vi "Set Exp to test_Charge Transfer.vi"(0 "Test Information":T3={"Exp Name"="Cold Switching", "Lot"="0233A", "Wafer"="15", "Die Type"="L22", "Die X "="6", "Die Y"="8", "Exp"="1", "Die X_Y"="8"}, 5 "Experiments":T2={"Exp 1"={"P2_Sweep_Stop_V"=36.0, "Res Threshold"=1.0, "P2_Sweep_Start_V"=36.0, "P2_Sweep_Step_V"=1.0, "Experiment Name"="", "P1_Sweep_Start_V"=36.0, "P1_Sweep_Step_V"=1.0, "P1_Peak_Array"=[]}, "Exp 2"={"P2_Sweep_Stop_V"=36.0, "Res Threshold"=1.0, "P2_Sweep_Start_V"=36.0, "P2_Sweep_Step_V"=1.0, "Experiment Name"="", "P1_Sweep_Start_V"=36.0, "P1_Sweep_Step_V"=1.0, "P1_Peak_Array"=[]}, "Exp 3"={"P2_Sweep_Stop_V"=36.0, "Res Threshold"=1.0, "P2_Sweep_Start_V"=36.0, "P2_Sweep_Step_V"=1.0, "Experiment Name"="", "P1_Sweep_Start_V"=36.0, "P1_Sweep_Step_V"=1.0, "P1_Peak_Array"=[]}, "Exp 4"={"P2_Sweep_Stop_V"=36.0, "Res Threshold"=1.0, "P2_Sweep_Start_V"=36.0, "P2_Sweep_Step_V"=1.0, "Experiment Name"="", "P1_Sweep_Start_V"=36.0, "P1_Sweep_Step_V"=1.0, "P1_Peak_Array"=[]}}, 11 "Error In":errorcluster) -> (4 "Selected Exp Settings":T1={"P2_Sweep_Stop_V"=36.0, "Res Threshold"=1.0, "P2_Sweep_Start_V"=36.0, "P2_Sweep_Step_V"=1.0, "Experiment Name"="", "P1_Sweep_Start_V"=36.0, "P1_Sweep_Step_V"=1.0, "P1_Peak_Array"=[10.0, 20.0, 30.0, 40.0]}, 6 "Test Information Out":T3={"Exp Name"="Cold Switching", "Lot"="0233A", "Wafer"="15", "Die Type"="L22", "Die X "="6", "Die Y"="8", "Exp"="1", "Die X_Y"="8"}, 15 "Error Out":errorcluster)   [LabVIEW 2013]
uses:
  Controls/Test Information.ctl
  Controls/Multiple Exp Setup_Charge Transfer.ctl
  Controls/Individual User Inputs_Charge Transfer.ctl
panel:
  # "Calc Settings"
  # "Test Settings"
  # "Calc Settings"
  # "Test Settings"
  # "Calc Settings"
  # "Test Settings"
  # "Calc Settings"
  # "Test Settings"
  # "Calc Settings"
  # "Test Settings"
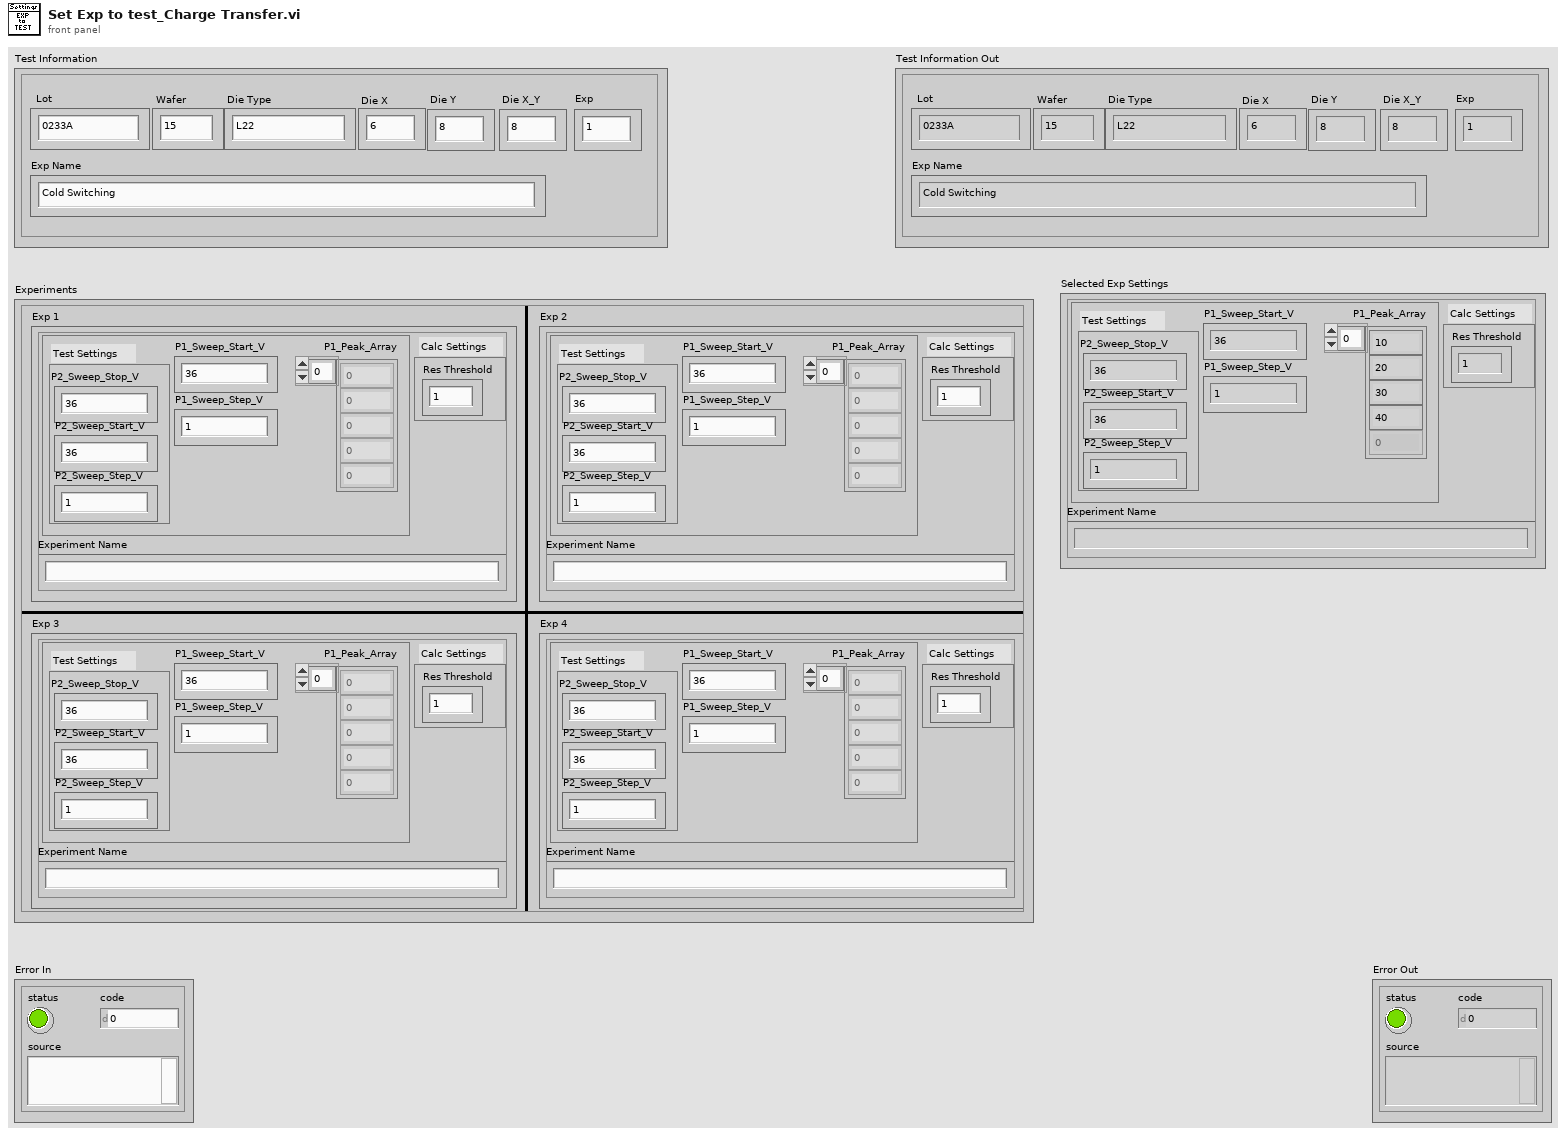
[diagram p1: front panel]
types:
  T1 = typedef "Individual User Inputs_Charge Transfer.ctl" = cluster{"P2_Sweep_Stop_V":dbl, "Res Threshold":dbl, "P2_Sweep_Start_V":dbl, "P2_Sweep_Step_V":dbl, "Experiment Name":string, "P1_Sweep_Start_V":dbl, "P1_Sweep_Step_V":dbl, "P1_Peak_Array":dbl[]}
  T2 = typedef "Multiple Exp Setup_Charge Transfer.ctl" = cluster{"Exp 1":T1, "Exp 2":T1, "Exp 3":T1, "Exp 4":T1}
  T3 = typedef "Test Information.ctl" = cluster{"Exp Name":string, "Lot":string, "Wafer":string, "Die Type":string, "Die X ":string, "Die Y":string, "Exp":string, "Die X_Y":string}
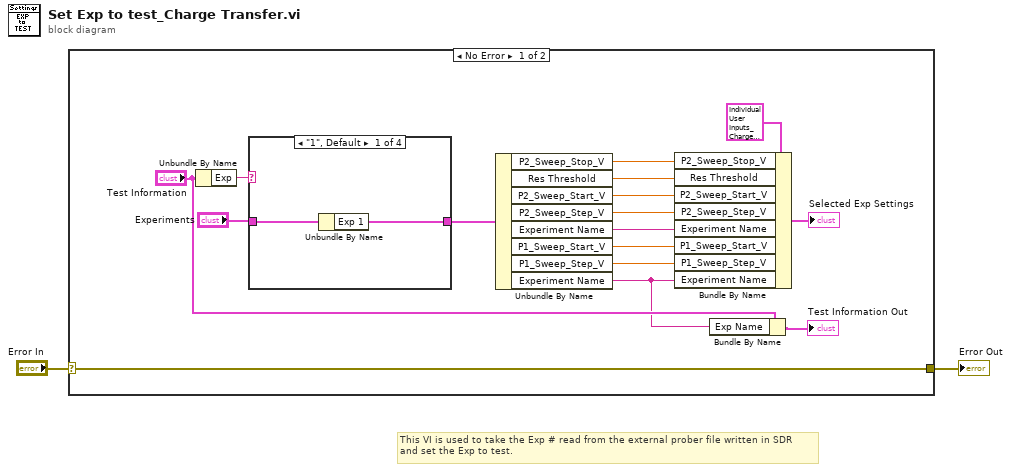
[diagram p0: block diagram]
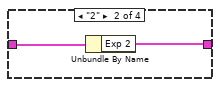
[diagram p2: hidden frame]
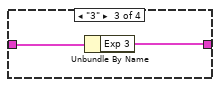
[diagram p3: hidden frame]
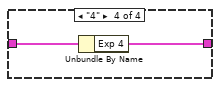
[diagram p4: hidden frame]
diagram:
  # "This VI is used to take the Exp # read from the external prober file written in SDR\nand set the Exp to test."
  n1 = case shown="No Error" "Error In" {
    selector: "Error In" -> [w6 w27]
    tunnel: [w6 w27] -> w1
    frame No Error {
      n2 = Unbundle By Name("Test Information") -> ("Exp"=w18:string)
      n3 = case shown="\"1\", Default" w18 {
        tunnel: [w19 w22 w24 w26] -> w15
        tunnel: "Experiments" -> [w20 w21 w23 w25]
        frame "1", Default {
          n4 = Unbundle By Name(w20) -> ("Exp 1"=w19:T1)
        }
        frame "2" {
          n5 = Unbundle By Name(w21) -> ("Exp 2"=w22:T1)
        }
        frame "3" {
          n6 = Unbundle By Name(w23) -> ("Exp 3"=w24:T1)
        }
        frame "4" {
          n7 = Unbundle By Name(w25) -> ("Exp 4"=w26:T1)
        }
      }
      n8 = Unbundle By Name(w15) -> ("P2_Sweep_Stop_V"=w14:dbl, "Res Threshold"=w13:dbl, "P2_Sweep_Start_V"=w12:dbl, "P2_Sweep_Step_V"=w11:dbl, "Experiment Name"=w4:string, "P1_Sweep_Start_V"=w10:dbl, "P1_Sweep_Step_V"=w9:dbl, "Experiment Name"=w8:string)
      n9 = Bundle By Name(cluster=T1 {"P2_Sweep_Stop_V"=36.0, "Res Threshold"=1.0, "P2_Sweep_Start_V"=36.0, "P2_Sweep_Step_V"=1.0, "Experiment Name"="", "P1_Sweep_Start_V"=36.0, "P1_Sweep_Step_V"=1.0, "P1_Peak_Array"=[10.0, 20.0, 30.0, 40.0]} ("Selected Exp Settings"), "P2_Sweep_Stop_V"=w14, "Res Threshold"=w13, "P2_Sweep_Start_V"=w12, "P2_Sweep_Step_V"=w11, "Experiment Name"=w4, "P1_Sweep_Start_V"=w10, "P1_Sweep_Step_V"=w9, "Experiment Name"=w8) -> (→"Selected Exp Settings":T1)
      n10 = Bundle By Name(cluster="Test Information", "Exp Name"=w8) -> (→"Test Information Out":T3)
    }
    frame Error {
    }
  }
  "Error Out" <- w1
